vi "Test VI.vi"   [LabVIEW 2019]
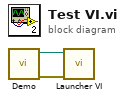
[diagram p0: block diagram]
diagram:
  n1 = call "Demo.vi"() -> ("error out"=w2:errorcluster, "directory copy"=w1:path)  [unwired: 10 in]
  n2 = call "Launcher VI.vi"("error in (no error)"=w2, "Folder Path"=w1) -> ()  [unwired: 9 in, 1 out]
